vi "TeleOp.vi"   [LabVIEW 2018]
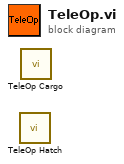
[diagram p0: block diagram]
diagram:
  n1 = call "TeleOp Hatch.vi"() -> ()  [unwired: 12 in]
  n2 = call "TeleOp Cargo.vi"() -> ()  [unwired: 12 in]
